vi "Test_Run All Tests.vi"(8 "error in":errorcluster, 9 "Modules":T7, 10 "Part Number 2":refnum<vi>, 11 "Test Selection":T8) -> (0 "error out":errorcluster)   [LabVIEW 2025]
uses:
  Controls/Test list.ctl
  Controls/tests tab control.ctl
  Controls/Graphs/XY Graph_Transparent.ctl
  Controls/Test Results/Test Pass Fail.ctl
  Controls/Test Results/Results Table.ctl
  Controls/Numeric Voltage.ctl
  Controls/Numeric Current.ctl
  SubVIs/Test_Calculate Wear-in.vi
  SubVIs/Test_Calculate Drop-out.vi
  SubVIs/Test_Calculate CRT.vi
  SubVIs/Test_Calculate Pull-in.vi
  SubVIs/Test_Calculate Hold-in.vi
  SubVIs/Test_Calculate ORT.vi
  Classes/Solenoid/Solenoid.lvclass
  Libraries/Power Supply/Power Supply.lvlib
  Libraries/USB IO/USB IO.lvlib
panel:
  out "Voltage Chart":dbl(graph)
  out "Current":T1 format="%5.3f A"
  out "Voltage":T2 format="%5.3f V"
  out "result 3":bool
  out "result 2":bool
  out "result":bool
  in  "Table Control":T3=[["Wear-in", "N/A", "N/A", "", "", "", "", ""], ["Drop-out", "N/A", "N/A", "", "", "", "", ""], ["Closing Response Time", "N/A", "N/A", "", "", "", "", ""], ["Pull-in", "N/A", "N/A", "", "", "", "", ""], ["Hold-in", "N/A", "N/A", "", "", "", "", ""], ["Opening Response Time", "N/A", "N/A", "", "", "", "", ""]]
  out "Errors":errorcluster
  in  "Tab Control":T4=enum."Wear-in"
  out "Power Supply Output":bool
  out "Cycles":dbl format="%3.0f of"
  out "Total Cycles":dbl format="%3.0f"
  out "Unit On?":bool
  in  "Abort":bool
  out "Drop-out Voltage":T2 format="%5.3f V"
  out "Drop-out Current":T1 format="%5.3f A"
  out "CRT Graph":T5
  out "Closing Response Time":dbl format="%5.3f ms"
  out "Pass? 2":T6 caption="Test Result"
  out "Pull-in Voltage":T2 format="%5.3f V"
  out "Pull-in Current":T1 format="%5.3f A"
  in  "Abort 2":bool
  out "XY Graph":T5
  out "Pass?":T6 caption="Test Result"
  out "Opening Response Time":dbl format="%5.3f ms"
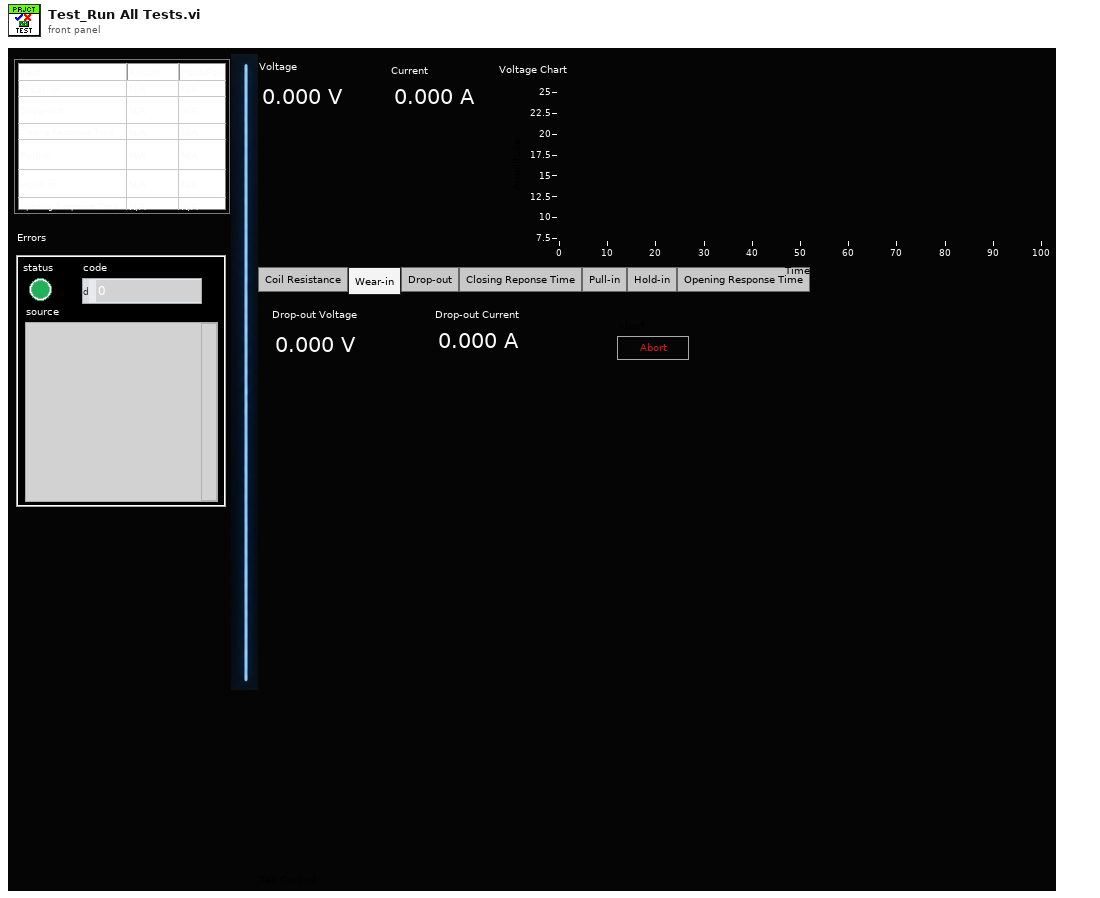
[diagram p1: front panel]
types:
  T1 = typedef "Numeric Current.ctl" = dbl
  T2 = typedef "Numeric Voltage.ctl" = dbl
  T3 = typedef "Results Table.ctl" = string[][]
  T4 = typedef "tests tab control.ctl" = enum32{"Coil Resistance", "Wear-in", "Drop-out", "Closing Reponse Time", "Pull-in", "Hold-in", "Opening Response Time"}
  T5 = typedef "XY Graph_Transparent.ctl" = cluster{dbl[], dbl[]}[]
  T6 = typedef "Test Pass Fail.ctl" = bool
  T7 = cluster{"Module IDs":i32[], "Module Names":string[]}
  T8 = typedef "Test list.ctl" = cluster{"Coil Resistance":bool, "Wear-in":bool, "Drop-out":bool, "Closing Response Time":bool, "Pull-in":bool, "Hold-in":bool, "Opening Response Time":bool}
  T9 = cluster{"V":dbl, "I":dbl, "Cycles":dbl, "On_Time_ms":dbl, "Off_Time_ms":dbl}
  T10 = cluster{"V":dbl, "I":dbl, "V_reduced":dbl, "V_perturb":dbl, "Plunger_Threshold":dbl, "Plunger_Threshold 2":dbl}
  T11 = cluster{"V":dbl, "I":dbl, "V_increased":dbl, "V_perturb":dbl, "Plunger_Threshold":dbl, "V_MAX":dbl}
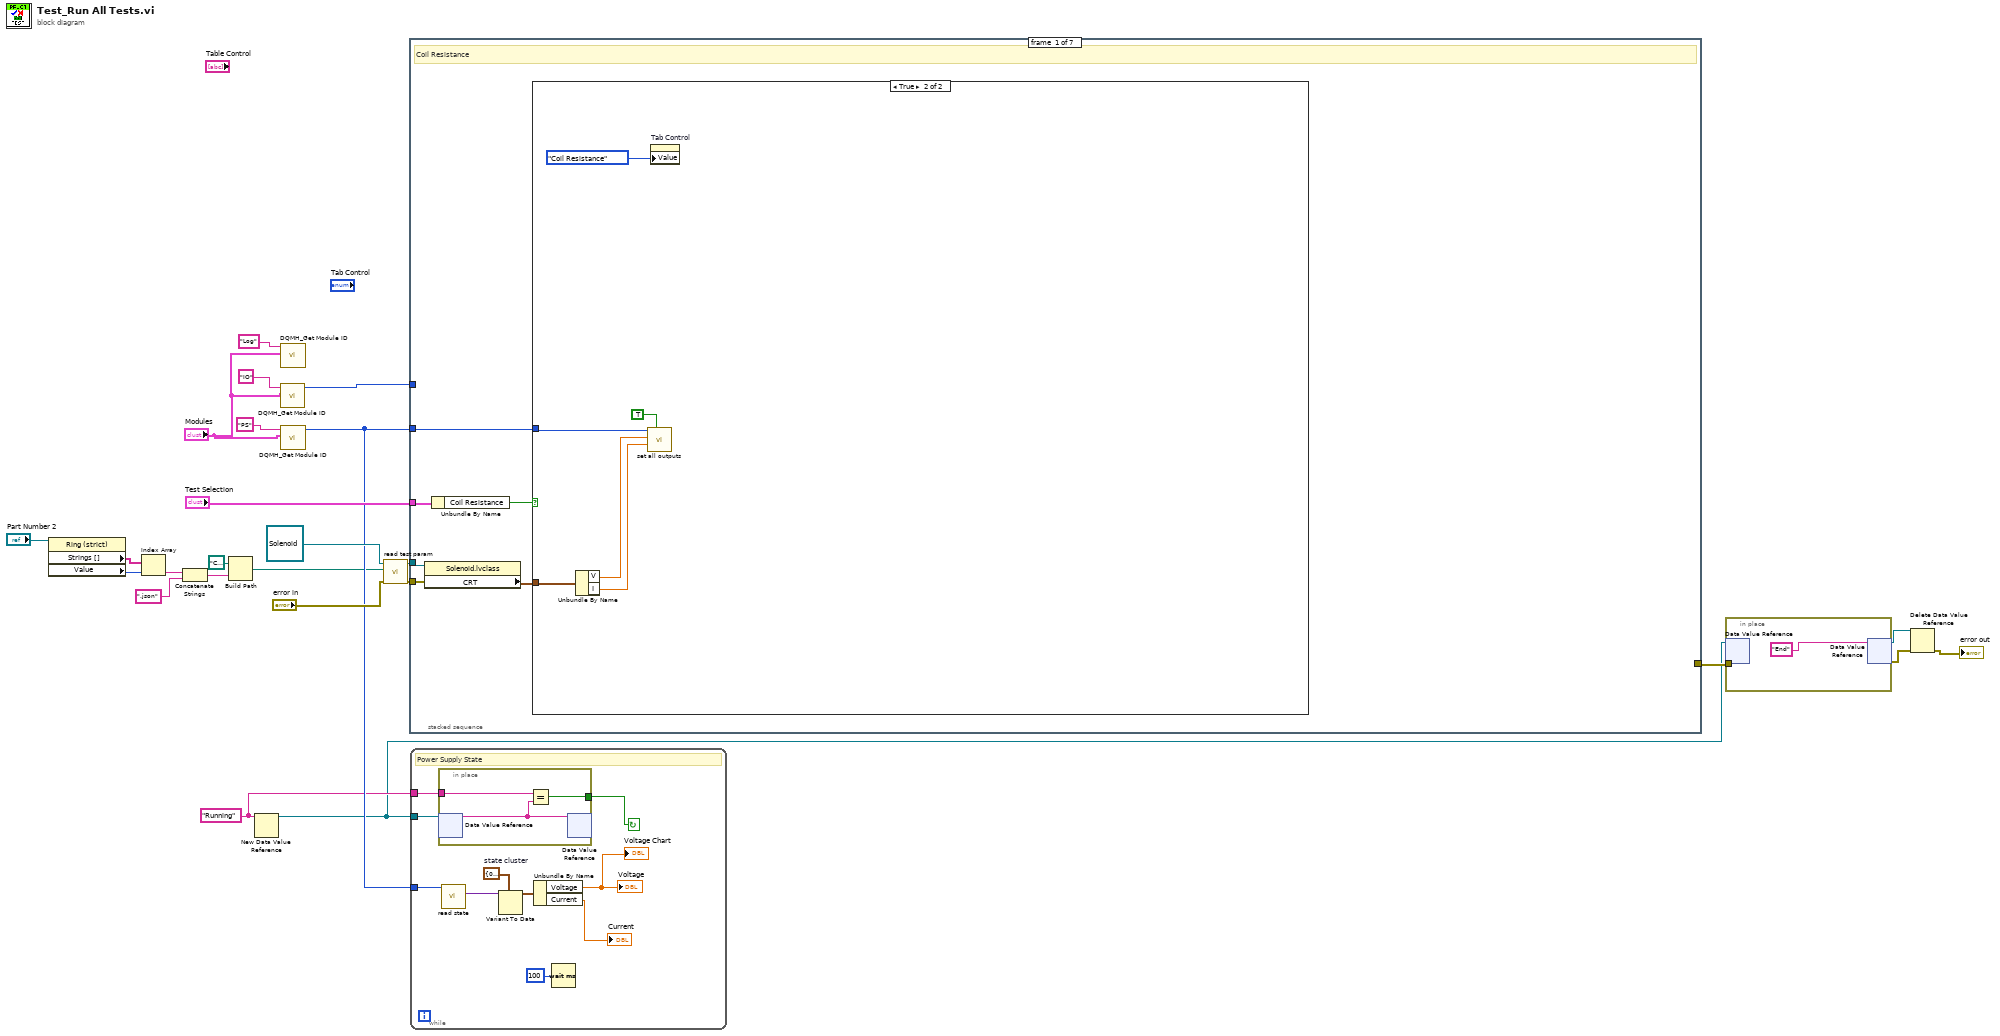
[diagram p0: block diagram]
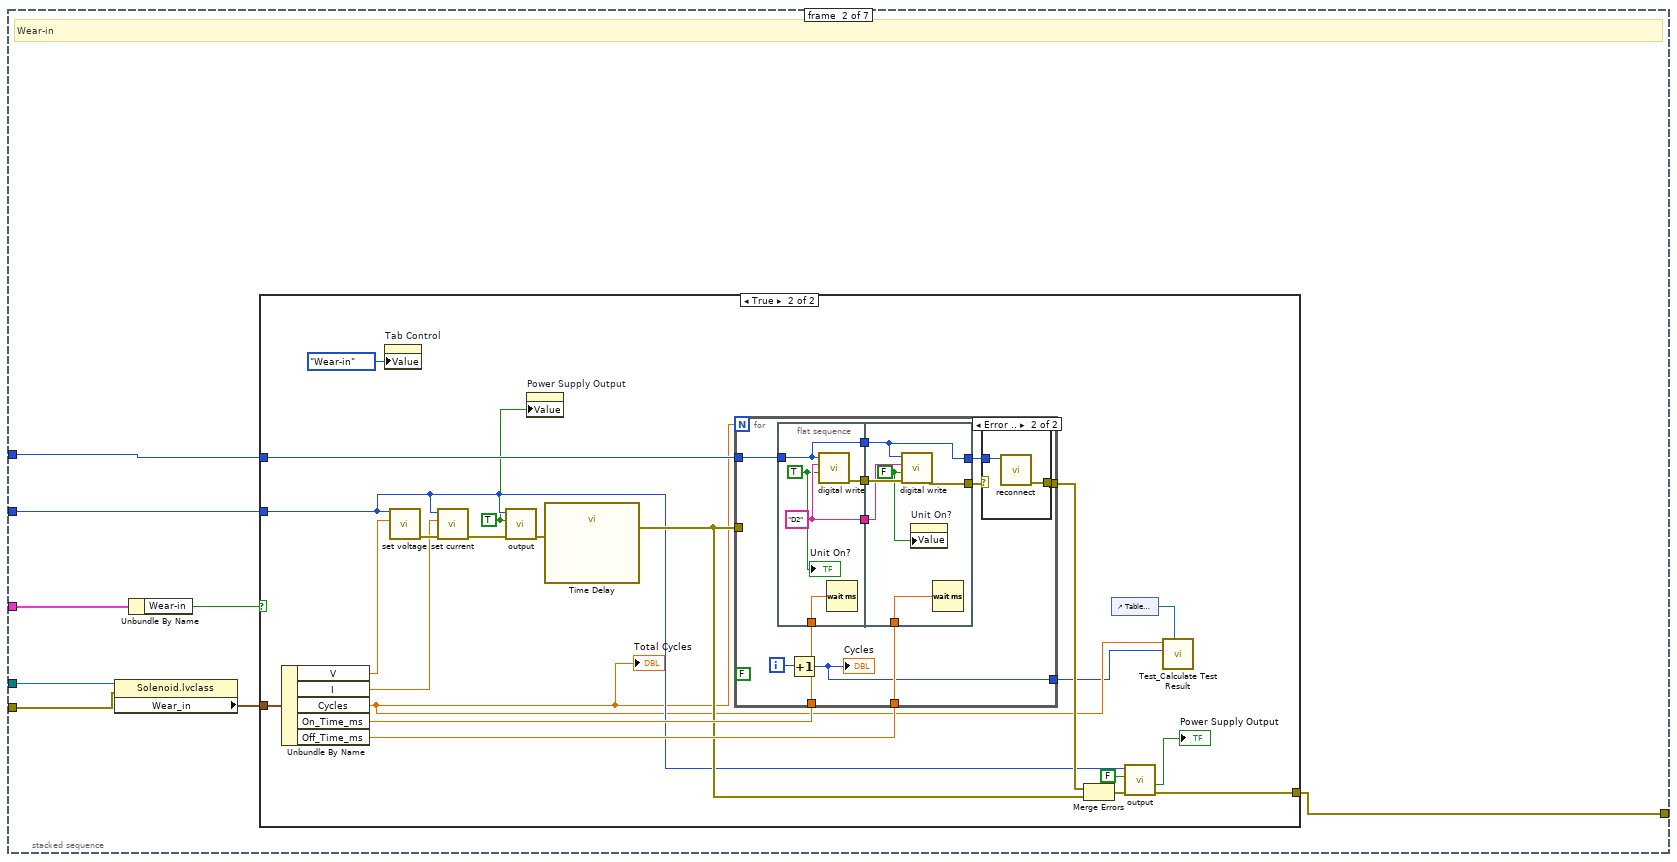
[diagram p3: hidden frame]
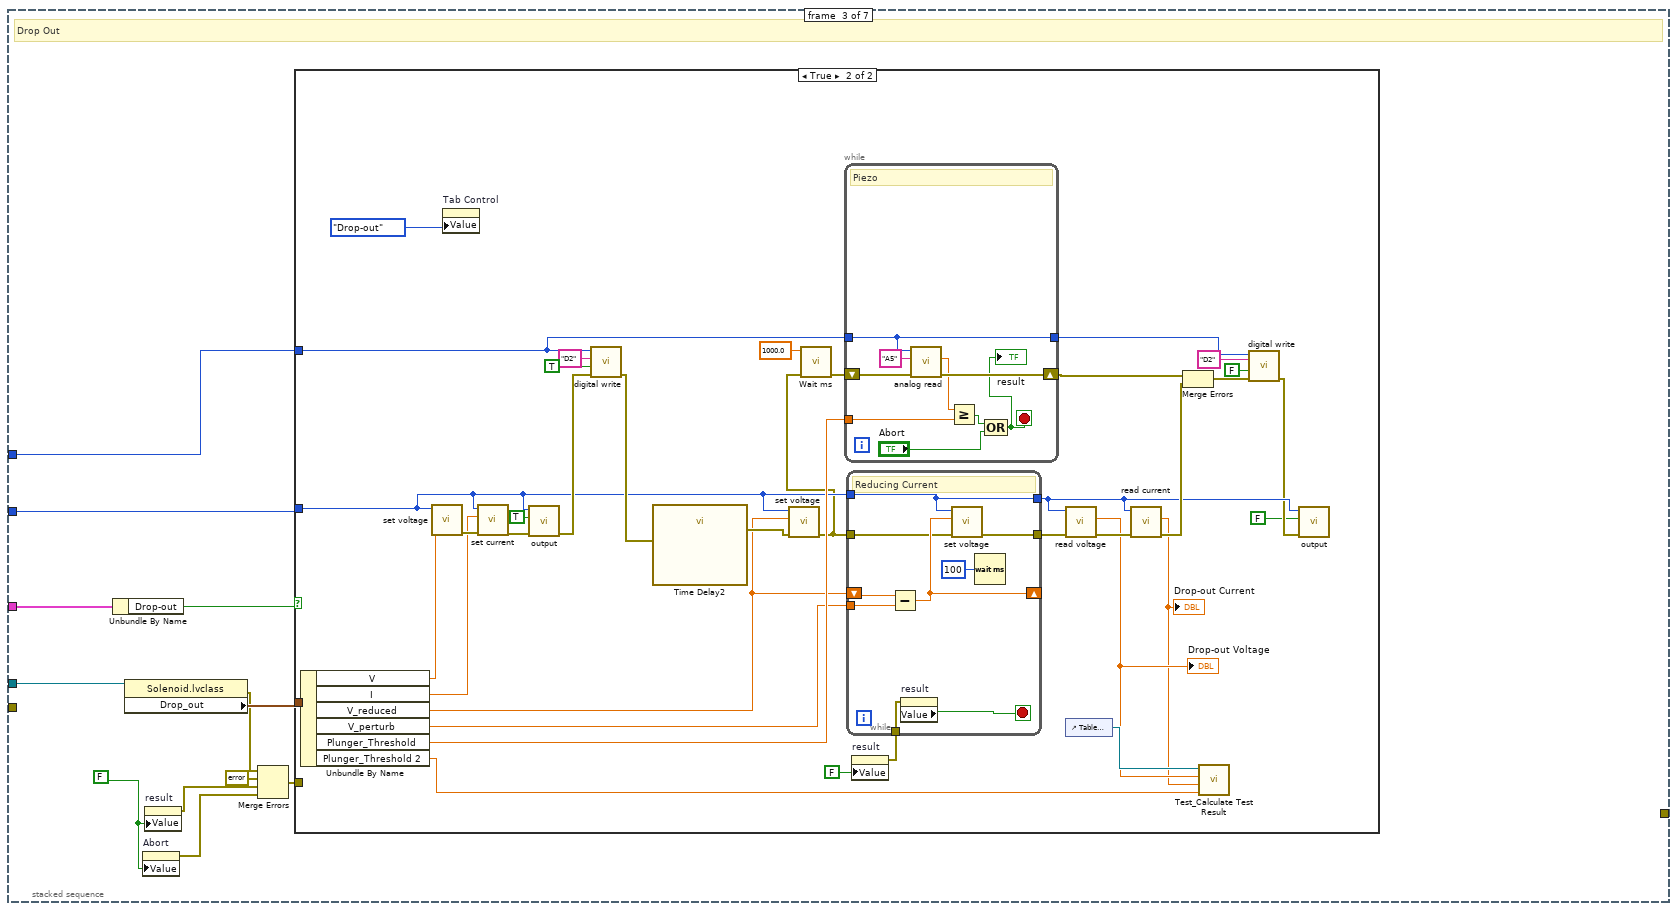
[diagram p6: hidden frame]
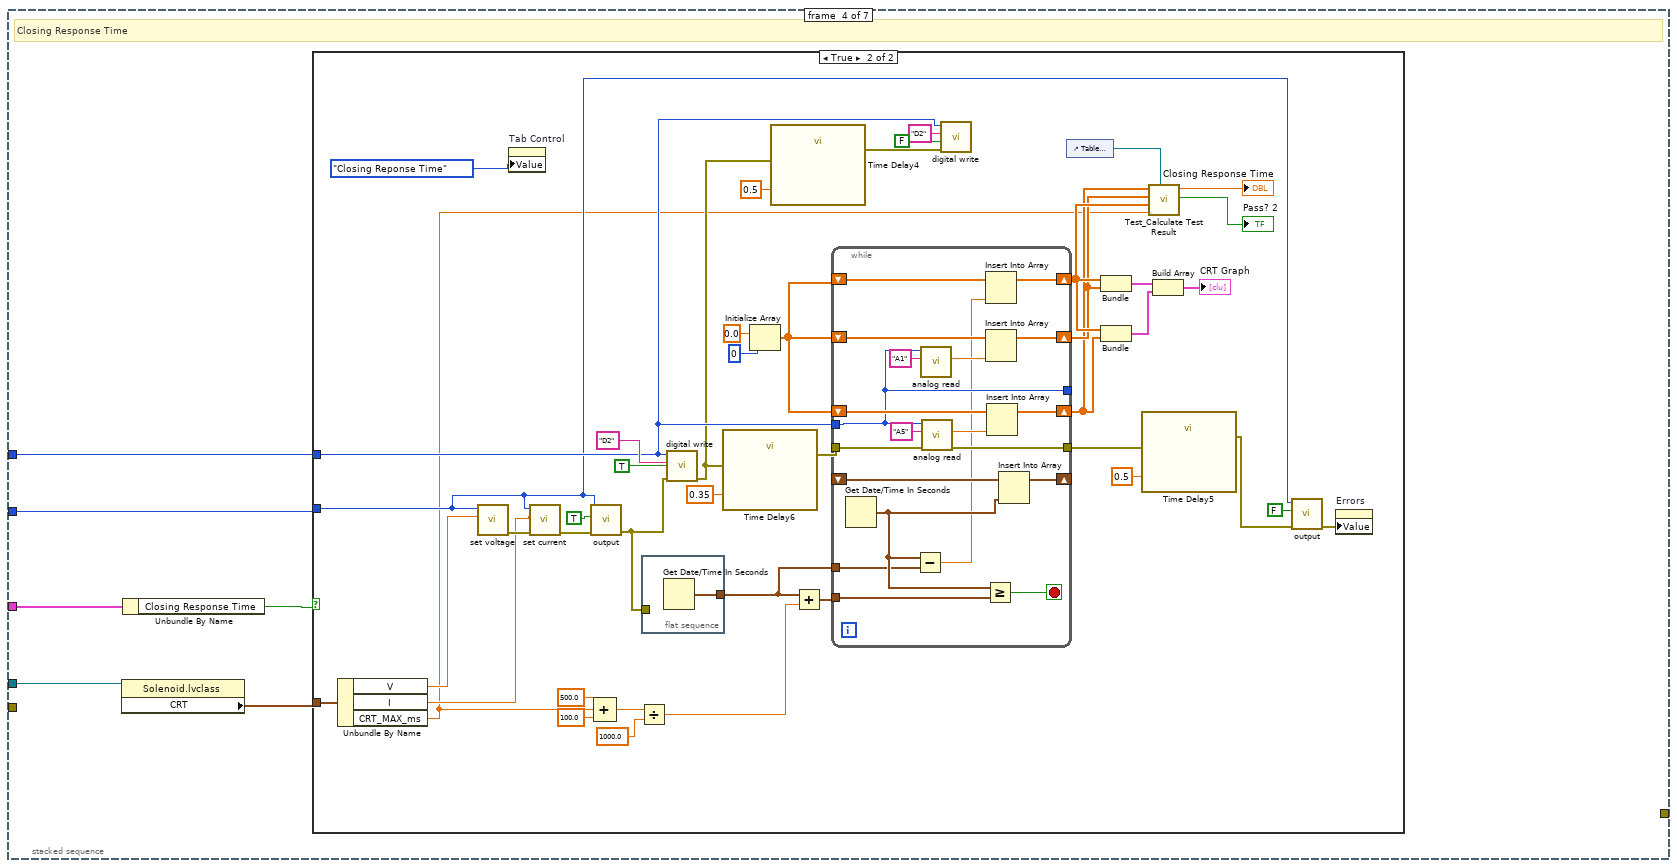
[diagram p8: hidden frame]
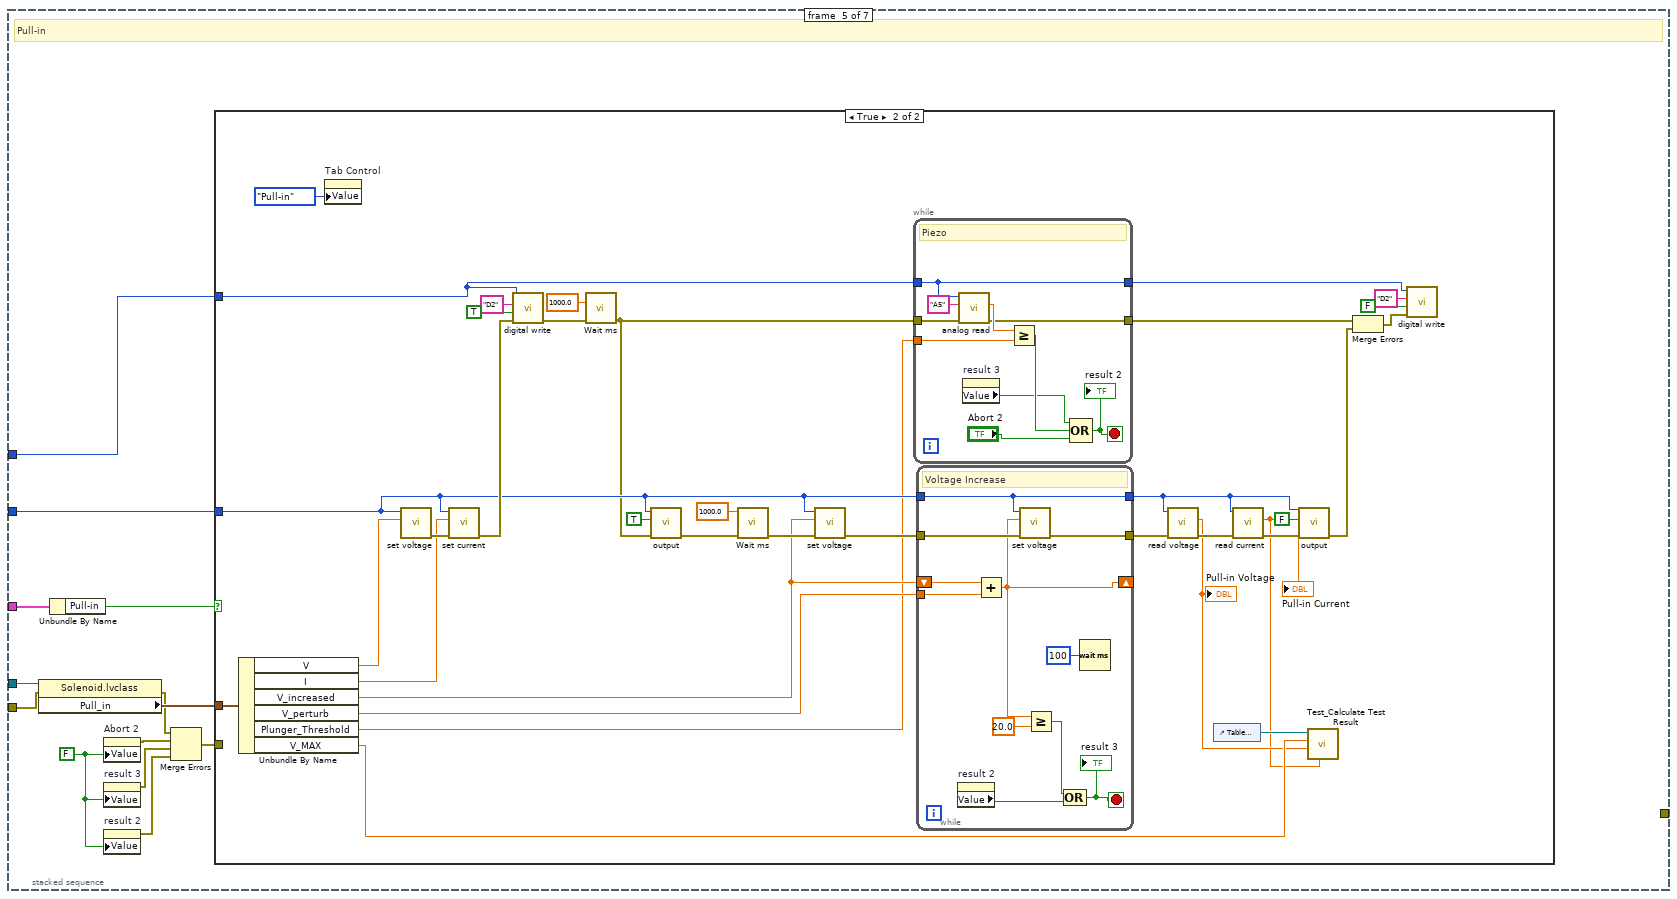
[diagram p10: hidden frame]
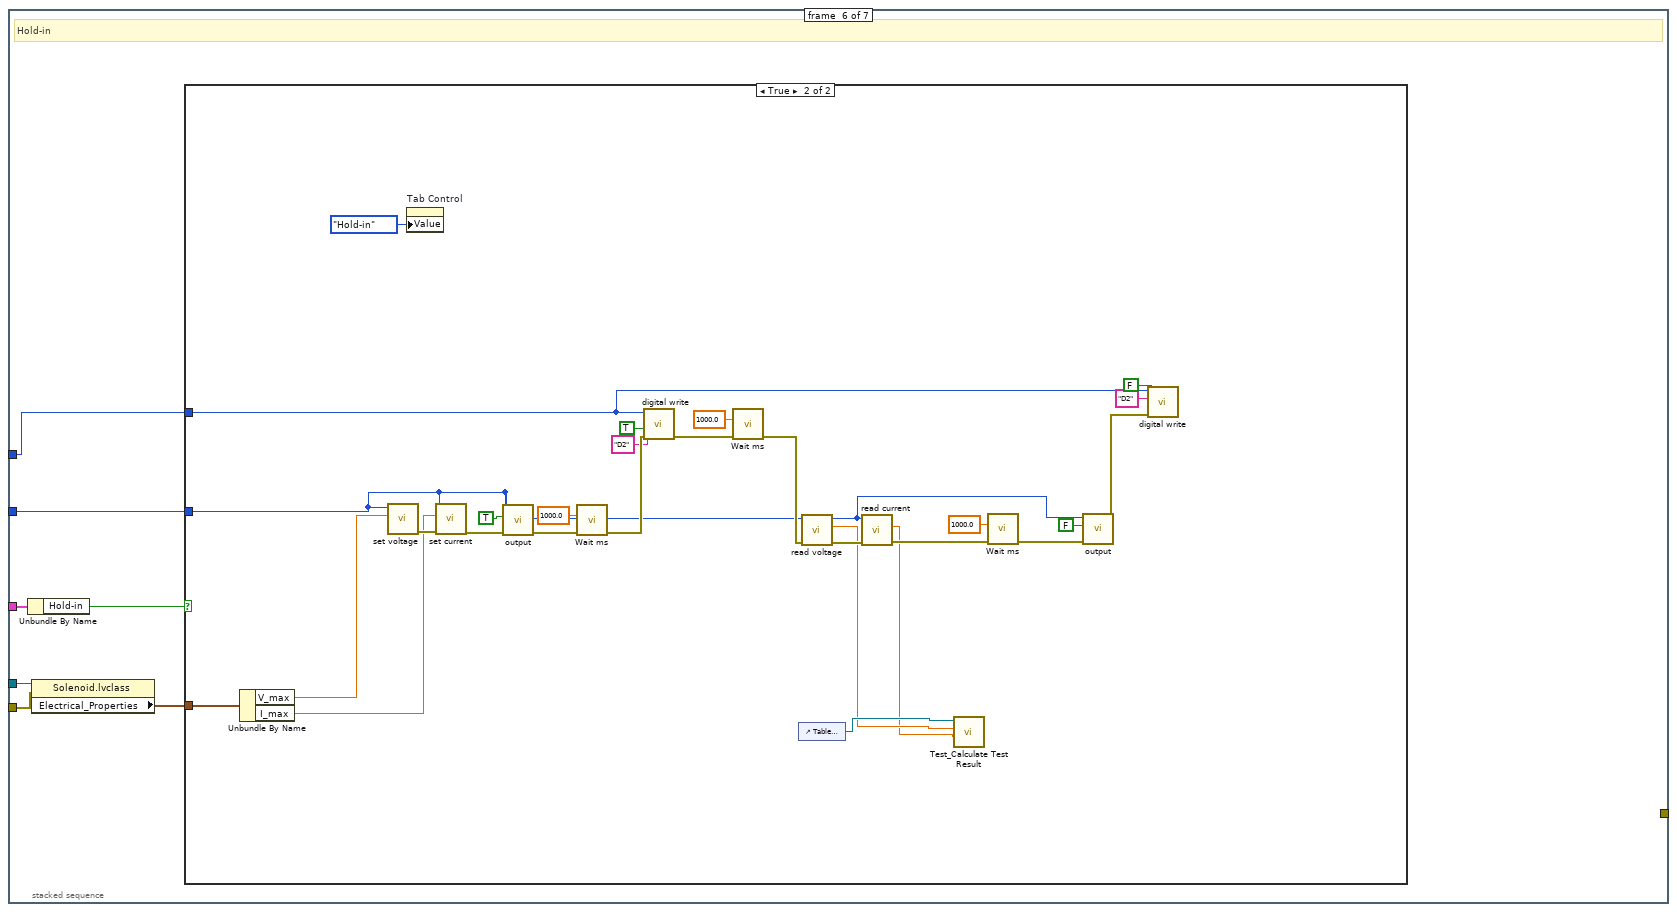
[diagram p12: hidden frame]
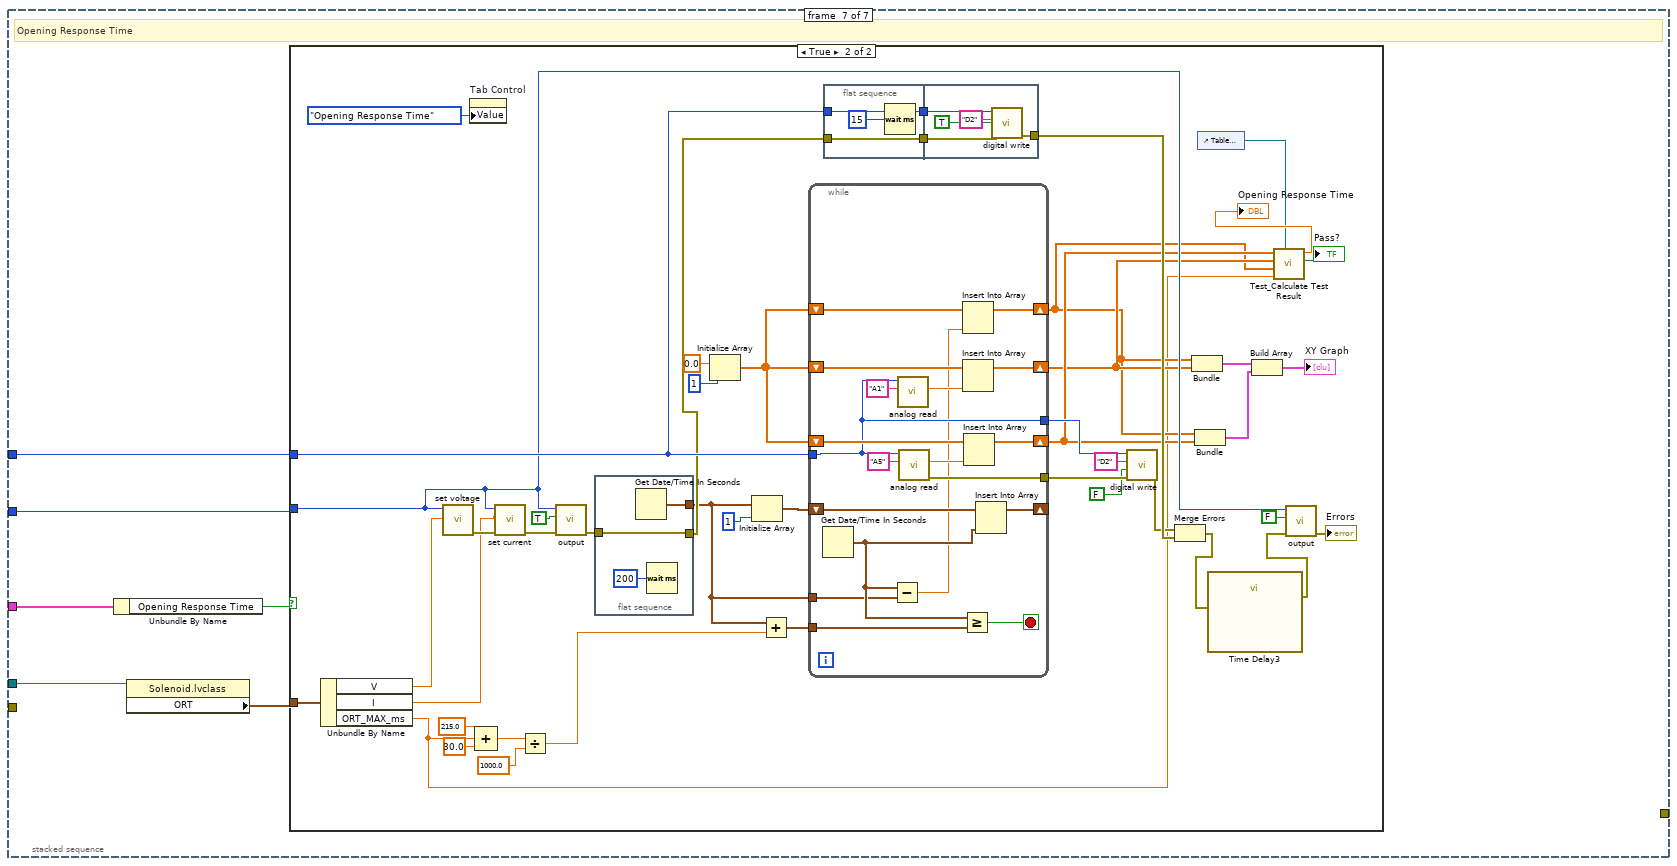
[diagram p14: hidden frame]
diagram:
  w14 = "Running"
  n1 = property class="Ring (strict)"(reference="Part Number 2") -> ("Strings []"=w7:string[], "Value"=w6:u16)  [unwired: 1 in, 2 out]
  n2 = Index Array(array=w7, index=w6) -> (element=w5:string)
  n3 = Concatenate Strings(w5, ".json" ("string")) -> (w3:string)
  n4 = Build Path(base path=path "C:/Users/Public/Documents/atp-station/programs", name or relative path=w3) -> (appended path=w1:path)
  n5 = New Data Value Reference(data value=w14) -> (data value reference=w12:refnum<data-value>)  [unwired: 1 in, 1 out]
  n6 = call "DQMH_Get Module ID.vi"("Modules"="Modules", "Module Name"="IO") -> ("Module ID out"=w16:i32)  [unwired: 9 in]
  n7 = call "DQMH_Get Module ID.vi"("Modules"="Modules", "Module Name"="Log") -> ()  [unwired: 9 in, 1 out]
  n8 = call "DQMH_Get Module ID.vi"("Modules"="Modules", "Module Name"="PS") -> ("Module ID out"=w15:i32)  [unwired: 9 in]
  n9 = call-dynamic "read test param.vi"("error in (no error)"="error in", "File Path"=w1, "Solenoid in"=refnum<class "Solenoid.lvclass"> refnum ("Solenoid.lvclass")) -> ("error out"=w21:errorcluster, "Solenoid out"=w23:refnum<class "Solenoid.lvclass">)  [unwired: 7 in]
  n10 = stacked-sequence {
    tunnel: w23 -> [w27 w43 w101 w162 w240 w304 w340]
    tunnel: "Test Selection" -> [w31 w45 w103 w164 w242 w306 w339]
    tunnel: w21 -> [w28 w42 _ _ w239 w303 _]
    tunnel: w15 -> [w29 w40 w99 w160 w237 w301 w336]
    tunnel: w16 -> [_ w39 w98 w159 w236 w300 w335]
    tunnel: [_ w38 _ _ _ _ _] -> w13
    frame #0 {
      # "Coil Resistance"
      n11 = property class="Solenoid.lvclass"(reference=w27, error in=w28) -> ("CRT"=w26:cluster{"V":dbl, "I":dbl, "CRT_MAX_ms":dbl})  [unwired: 2 out]
      n12 = Unbundle By Name(w31) -> ("Coil Resistance"=w30:bool)
      n13 = case shown="True" w30 {
        tunnel: w29 -> [_ w36]
        tunnel: w26 -> [_ w35]
        frame False {
        }
        frame True {
          n14 = Unbundle By Name(w35) -> ("V"=w33:dbl, "I"=w32:dbl)
          n15 = call "set all outputs.vi"("Output On/Off"=TRUE, "Current"=w32, "Voltage"=w33, "Module ID"=w36) -> ()  [unwired: 6 in, 2 out]
          n16 = property on="Tab Control" class="TabCtl (strict)"("Value"=tests_tab_control."Coil Resistance" ("Tab Control")) -> ()  [unwired: 2 in, 2 out]
        }
      }
    }
    frame #1 {
      # "Wear-in"
      n17 = property class="Solenoid.lvclass"(reference=w43, error in=w42) -> ("Wear_in"=w41:T9)  [unwired: 2 out]
      n18 = Unbundle By Name(w45) -> ("Wear-in"=w44:bool)
      n19 = case shown="True" w44 {
        tunnel: w41 -> [_ w66]
        tunnel: w40 -> [_ w55]
        tunnel: w39 -> [_ w62]
        tunnel: [_ w56] -> w38
        frame False {
        }
        frame True {
          w53 = TRUE ("Output On/Off")
          n20 = Unbundle By Name(w66) -> ("V"=w48:dbl, "I"=w47:dbl, "Cycles"=w51:dbl, "On_Time_ms"=w64:dbl, "Off_Time_ms"=w63:dbl)
          "Total Cycles" <- w51
          n21 = property on="Tab Control" class="TabCtl (strict)"("Value"=tests_tab_control."Wear-in" ("Tab Control")) -> ()  [unwired: 2 in, 2 out]
          n22 = call "set voltage.vi"("Output Voltage"=w48, "Module ID"=w55) -> ("error out"=w65:errorcluster)  [unwired: 8 in, 1 out]
          n23 = call "set current.vi"("error in"=w65, "Output Current"=w47, "Module ID"=w55) -> ("error out"=w61:errorcluster)  [unwired: 7 in, 1 out]
          n24 = call "output.vi"("error in"=w61, "Output On/Off"=w53, "Module ID"=w55) -> ("error out"=w60:errorcluster)  [unwired: 7 in, 1 out]
          n25 = property on="Power Supply Output" class="Bool (strict)"("Value"=w53) -> ()  [unwired: 2 in, 2 out]
          n26 = call "Time Delay"("error in (no error)"=w60) -> ("error out"=w58:errorcluster)  [unwired: 10 in]
          n27 = for {
            N: w51 -> [_]
            tunnel: w64 -> [w77]
            tunnel: w63 -> [w76]
            tunnel: w62 -> [w75]
            tunnel: w58 -> [_]
            tunnel: [w69] -> w59
            tunnel: [w67] -> w50
            i -> [w71]
            (unwired) FALSE ("Power Supply Output")
            n28 = flat-sequence {
              tunnel: w77 -> [w85]
              tunnel: w75 -> [w83]
              tunnel: [w84] -> w74
              tunnel: [w83] -> w73
              tunnel: [w82] -> w72
              tunnel: w76 -> [w89]
              tunnel: w74 -> [w91]
              tunnel: w73 -> [w86]
              tunnel: w72 -> [w90]
              tunnel: [w88] -> w70
              tunnel: [w86] -> w68
              frame #0 {
                w81 = TRUE ("On/Off")
                w82 = "D2" ("Line")
                n29 = call "digital write.vi"("On/Off"=w81, "Line"=w82, "Module ID"=w83) -> ("error out"=w84:errorcluster)  [unwired: 7 in, 1 out]
                n30 = Wait (ms)(milliseconds to wait=w85) -> ()  [unwired: 1 out]
                "Unit On?" <- w81
              }
              frame #1 {
                w87 = FALSE ("On/Off")
                n31 = call "digital write.vi"("error in"=w91, "On/Off"=w87, "Line"=w90, "Module ID"=w86) -> ("error out"=w88:errorcluster)  [unwired: 6 in, 1 out]
                n32 = property on="Unit On?" class="Bool (strict)"("Value"=w87) -> ()  [unwired: 2 in, 2 out]
                n33 = Wait (ms)(milliseconds to wait=w89) -> ()  [unwired: 1 out]
              }
            }
            n34 = Increment(x=w71) -> (x+1=w67:i32)
            "Cycles" <- w67
            n35 = case shown="Error .." w70 {
              selector: w70 -> [w78 _]
              tunnel: [w78 w80] -> w69
              tunnel: w68 -> [_ w79]
              frame No Error {
              }
              frame Error {
                n36 = call "reconnect.vi"("Module ID"=w79) -> ("error out"=w80:errorcluster)  [unwired: 9 in, 1 out]
              }
            }
          }
          n37 = Merge Errors(w59, w58) -> (w57:errorcluster)
          n38 = control-ref of="Table Control"() -> (w49:refnum<vi>)
          n39 = call "output.vi"("error in"=w57, "Output On/Off"=FALSE, "Module ID"=w55) -> ("error out"=w56:errorcluster, "timed out?"=→"Power Supply Output":bool)  [unwired: 7 in]
          n40 = call-poly "Test_Calculate Test Result.vi"("Table Ref"=w49, "Cycles"=w50, "Total Cycles"=w51) -> ()  [unwired: 7 in, 2 out]
        }
      }
    }
    frame #2 {
      w97 = FALSE
      # "Drop Out"
      n41 = Unbundle By Name(w103) -> ("Drop-out"=w102:bool)
      n42 = property class="Solenoid.lvclass"(reference=w101) -> (error out=w96:errorcluster, "Drop_out"=w100:T10)  [unwired: 1 in, 1 out]
      n43 = property on="Abort" class="Bool (strict)"("Value"=w97) -> (error out=w94:errorcluster)  [unwired: 2 in, 1 out]
      n44 = property on="result" class="Bool (strict)"("Value"=w97) -> (error out=w95:errorcluster)  [unwired: 2 in, 1 out]
      n45 = Merge Errors(w96, errorcluster {"status"=FALSE, "code"=0, "source"=""} ("error in"), w95, w94) -> (w93:errorcluster)
      n46 = case shown="True" w102 {
        tunnel: w100 -> [_ w140]
        tunnel: w99 -> [_ w127]
        tunnel: w98 -> [_ w131]
        tunnel: w93 -> [_ _]
        frame False {
        }
        frame True {
          n47 = Unbundle By Name(w140) -> ("V"=w106:dbl, "I"=w105:dbl, "V_reduced"=w129:dbl, "V_perturb"=w128:dbl, "Plunger_Threshold"=w130:dbl, "Plunger_Threshold 2"=w112:dbl)
          n48 = call "set voltage.vi"("Output Voltage"=w106, "Module ID"=w127) -> ("error out"=w139:errorcluster)  [unwired: 8 in, 1 out]
          n49 = property on="Tab Control" class="TabCtl (strict)"("Value"=tests_tab_control."Drop-out" ("Tab Control")) -> ()  [unwired: 2 in, 2 out]
          n50 = call "set current.vi"("error in"=w139, "Output Current"=w105, "Module ID"=w127) -> ("error out"=w138:errorcluster)  [unwired: 7 in, 1 out]
          n51 = call "output.vi"("error in"=w138, "Output On/Off"=TRUE, "Module ID"=w127) -> ("error out"=w136:errorcluster)  [unwired: 7 in, 1 out]
          n52 = call "digital write.vi"("error in"=w136, "On/Off"=TRUE, "Line"="D2", "Module ID"=w131) -> ("error out"=w132:errorcluster)  [unwired: 6 in, 1 out]
          n53 = call "Time Delay2"("error in (no error)"=w132) -> ("error out"=w133:errorcluster)  [unwired: 10 in]
          n54 = call "set voltage.vi"("error in"=w133, "Output Voltage"=w129, "Module ID"=w127) -> ("error out"=w110:errorcluster)  [unwired: 7 in, 1 out]
          n55 = call "Wait ms.vi"("error in (no error)"=w110, "Delay Time (ms)"=1000.0) -> ("error out"=w111:errorcluster)  [unwired: 9 in]
          n56 = while {
            tunnel: w131 -> [w154]
            shift-right: [w157] -> w124
            shift-left: w111 -> [w151]
            tunnel: w130 -> [w155]
            tunnel: [w154] -> w122
            stop <- w152 stop-if-true
            # "Piezo"
            n57 = call "analog read.vi"("error in"=w151, "Line"="A5", "Module ID"=w154) -> ("error out"=w157:errorcluster, "Voltage"=w156:T2)  [unwired: 6 in, 1 out]
            n58 = Greater Or Equal?(x=w156, y=w155) -> (x >= y?=w150:bool)
            n59 = Compound Arithmetic op=OR(w150, "Abort") -> (w152:bool)
            "result" <- w152
          }
          n60 = property on="result" class="Bool (strict)"("Value"=FALSE) -> (error out=w108:errorcluster)  [unwired: 2 in, 1 out]
          n61 = while {
            shift-right: [w144] -> _
            shift-left: w129 -> [w149]
            tunnel: w128 -> [w148]
            tunnel: w110 -> [w143]
            tunnel: w127 -> [w145]
            tunnel: [w147] -> w126
            tunnel: [w145] -> w119
            tunnel: w108 -> [w142]
            stop <- w141 stop-if-true
            # "Reducing Current"
            n62 = Subtract(x=w149, y=w148) -> (x-y=w144:dbl)
            n63 = property on="result" class="Bool (strict)"(error in=w142) -> ("Value"=w141:bool)  [unwired: 1 in, 2 out]
            n64 = call "set voltage.vi"("error in"=w143, "Output Voltage"=w144, "Module ID"=w145) -> ("error out"=w147:errorcluster)  [unwired: 7 in, 1 out]
            n65 = Wait (ms)(milliseconds to wait=u32 100) -> ()  [unwired: 1 out]
          }
          n66 = call "read voltage.vi"("error in"=w126, "Module ID"=w119) -> ("error out"=w125:errorcluster, "Volts"=w114:T2)  [unwired: 7 in, 1 out]
          "Drop-out Voltage" <- w114
          n67 = control-ref of="Table Control"() -> (w115:refnum<vi>)
          n68 = call "read current.vi"("error in"=w125, "Module ID"=w119) -> ("error out"=w123:errorcluster, "Amps"=w113:T1)  [unwired: 7 in, 1 out]
          "Drop-out Current" <- w113
          n69 = Merge Errors(w124, w123) -> (w118:errorcluster)
          n70 = call-poly "Test_Calculate Test Result.vi"("V_MIN"=w112, "Amps"=w113, "Volts"=w114, "Table in"=w115) -> ()  [unwired: 8 in]
          n71 = call "digital write.vi"("error in"=w118, "On/Off"=FALSE, "Line"="D2", "Module ID"=w122) -> ("error out"=w117:errorcluster)  [unwired: 6 in, 1 out]
          n72 = call "output.vi"("error in"=w117, "Output On/Off"=FALSE, "Module ID"=w119) -> ()  [unwired: 7 in, 2 out]
        }
      }
    }
    frame #3 {
      # "Closing Response Time"
      n73 = property class="Solenoid.lvclass"(reference=w162) -> ("CRT"=w161:cluster{"V":dbl, "I":dbl, "CRT_MAX_ms":dbl})  [unwired: 1 in, 2 out]
      n74 = Unbundle By Name(w164) -> ("Closing Response Time"=w163:bool)
      n75 = case shown="True" w163 {
        tunnel: w161 -> [_ w208]
        tunnel: w160 -> [_ w180]
        tunnel: w159 -> [_ w185]
        frame False {
        }
        frame True {
          n76 = Unbundle By Name(w208) -> ("V"=w203:dbl, "I"=w204:dbl, "CRT_MAX_ms"=w170:dbl)
          n77 = call "set voltage.vi"("Output Voltage"=w203, "Module ID"=w180) -> ("error out"=w207:errorcluster)  [unwired: 8 in, 1 out]
          n78 = property on="Tab Control" class="TabCtl (strict)"("Value"=tests_tab_control."Closing Reponse Time" ("Tab Control")) -> ()  [unwired: 2 in, 2 out]
          n79 = call "set current.vi"("error in"=w207, "Output Current"=w204, "Module ID"=w180) -> ("error out"=w205:errorcluster)  [unwired: 7 in, 1 out]
          n80 = call "output.vi"("error in"=w205, "Output On/Off"=TRUE, "Module ID"=w180) -> ("error out"=w200:errorcluster)  [unwired: 7 in, 1 out]
          n81 = Compound Arithmetic op=ADD(500.0 ("value"), w170, 100.0 ("value")) -> (w197:dbl)
          n82 = Divide(x=w197, y=1000.0) -> (x/y=w193:dbl)
          n83 = flat-sequence {
            tunnel: w200 -> [_]
            tunnel: [w209] -> w194
            frame #0 {
              n84 = Get Date/Time In Seconds() -> (seconds since 1Jan1904=w209:timestamp)
            }
          }
          n85 = call "digital write.vi"("error in"=w200, "On/Off"=TRUE, "Line"="D2", "Module ID"=w185) -> ("error out"=w175:errorcluster)  [unwired: 6 in, 1 out]
          n86 = call "Time Delay6"("error in (no error)"=w175, "Delay Time (s)"=0.35) -> ("error out"=w174:errorcluster)  [unwired: 9 in]
          n87 = Initialize Array(0.0 ("element"), 0 ("dimension size")) -> (w190:dbl[])
          n88 = call "Time Delay4"("error in (no error)"=w175, "Delay Time (s)"=0.5) -> ("error out"=w188:errorcluster)  [unwired: 9 in]
          n89 = Add(x=w194, y=w193) -> (x+y=w195:timestamp)
          n90 = while {
            shift-right: [w222] -> w172
            shift-left: w190 -> [w229]
            shift-right: [w227] -> w171
            shift-left: w190 -> [w226]
            tunnel: w185 -> [w220]
            tunnel: [w221] -> w184
            tunnel: [w220] -> _
            shift-right: [w218] -> _
            shift-left: _ -> [w219]
            tunnel: w195 -> [w215]
            shift-right: [w214] -> w173
            shift-left: w190 -> [w213]
            tunnel: w194 -> [w211]
            tunnel: w174 -> [w210]
            stop <- w217 stop-if-true
            n91 = Get Date/Time In Seconds() -> (seconds since 1Jan1904=w216:timestamp)
            n92 = Subtract(x=w216, y=w211) -> (x-y=w212:dbl)
            n93 = call "analog read.vi"("Line"="A1", "Module ID"=w220) -> ("Voltage"=w228:T2)  [unwired: 7 in, 2 out]
            n94 = call "analog read.vi"("error in"=w210, "Line"="A5", "Module ID"=w220) -> ("error out"=w221:errorcluster, "Voltage"=w225:T2)  [unwired: 6 in, 1 out]
            n95 = Greater Or Equal?(x=w216, y=w215) -> (x >= y?=w217:bool)
            n96 = Insert Into Array(array=w213, new element=w212) -> (w214:dbl[])  [unwired: 1 in]
            n97 = Insert Into Array(array=w229, new element=w228) -> (w222:dbl[])  [unwired: 1 in]
            n98 = Insert Into Array(array=w226, new element=w225) -> (w227:dbl[])  [unwired: 1 in]
            n99 = Insert Into Array(array=w219, new element=w216) -> (w218:timestamp[])  [unwired: 1 in]
          }
          n100 = call "digital write.vi"("error in"=w188, "On/Off"=FALSE, "Line"="D2", "Module ID"=w185) -> ()  [unwired: 6 in, 2 out]
          n101 = control-ref of="Table Control"() -> (w166:refnum<vi>)
          n102 = Bundle(w173, w172) -> (w178:cluster{dbl[], dbl[]})  [unwired: 1 in]
          n103 = Bundle(w173, w171) -> (w177:cluster{dbl[], dbl[]})  [unwired: 1 in]
          n104 = call "Time Delay5"("error in (no error)"=w184, "Delay Time (s)"=0.5) -> ("error out"=w182:errorcluster)  [unwired: 9 in]
          n105 = call-poly "Test_Calculate Test Result.vi"("Table Ref"=w166, "CRT_MAX"=w170, "Time Data"=w173, "Current Data"=w172, "Piezo Data"=w171) -> ("Pass?"=→"Pass? 2":bool, "CRT [ms]"=→"Closing Response Time":dbl)  [unwired: 5 in]
          n106 = Build Array(w178, w177) -> (→"CRT Graph":cluster{dbl[], dbl[]}[])
          n107 = call "output.vi"("error in"=w182, "Output On/Off"=FALSE, "Module ID"=w180) -> ("error out"=w179:errorcluster)  [unwired: 7 in, 1 out]
          n108 = property on="Errors" class="Clust (strict)"("Value"=w179) -> ()  [unwired: 2 in, 2 out]
        }
      }
    }
    frame #4 {
      w231 = FALSE
      # "Pull-in"
      n109 = property class="Solenoid.lvclass"(reference=w240, error in=w239) -> (error out=w235:errorcluster, "Pull_in"=w238:T11)  [unwired: 1 out]
      n110 = Unbundle By Name(w242) -> ("Pull-in"=w241:bool)
      n111 = property on="Abort 2" class="Bool (strict)"("Value"=w231) -> (error out=w234:errorcluster)  [unwired: 2 in, 1 out]
      n112 = property on="result 3" class="Bool (strict)"("Value"=w231) -> (error out=w233:errorcluster)  [unwired: 2 in, 1 out]
      n113 = property on="result 2" class="Bool (strict)"("Value"=w231) -> (error out=w232:errorcluster)  [unwired: 2 in, 1 out]
      n114 = Merge Errors(w235, w234, w233, w232) -> (w230:errorcluster)
      n115 = case shown="True" w241 {
        tunnel: w238 -> [_ w276]
        tunnel: w237 -> [_ w263]
        tunnel: w236 -> [_ w261]
        tunnel: w230 -> [_ _]
        frame False {
        }
        frame True {
          n116 = Unbundle By Name(w276) -> ("V"=w275:dbl, "I"=w244:dbl, "V_increased"=w266:dbl, "V_perturb"=w265:dbl, "Plunger_Threshold"=w260:dbl, "V_MAX"=w247:dbl)
          n117 = property on="Tab Control" class="TabCtl (strict)"("Value"=tests_tab_control."Pull-in" ("Tab Control")) -> ()  [unwired: 2 in, 2 out]
          n118 = call "set voltage.vi"("Output Voltage"=w275, "Module ID"=w263) -> ("error out"=w278:errorcluster)  [unwired: 8 in, 1 out]
          n119 = call "set current.vi"("error in"=w278, "Output Current"=w244, "Module ID"=w263) -> ("error out"=w272:errorcluster)  [unwired: 7 in, 1 out]
          n120 = call "digital write.vi"("error in"=w272, "On/Off"=TRUE, "Line"="D2", "Module ID"=w261) -> ("error out"=w271:errorcluster)  [unwired: 6 in, 1 out]
          n121 = call "Wait ms.vi"("error in (no error)"=w271, "Delay Time (ms)"=1000.0) -> ("error out"=w262:errorcluster)  [unwired: 9 in]
          n122 = call "output.vi"("error in"=w262, "Output On/Off"=TRUE, "Module ID"=w263) -> ("error out"=w269:errorcluster)  [unwired: 7 in, 1 out]
          n123 = call "Wait ms.vi"("error in (no error)"=w269, "Delay Time (ms)"=1000.0) -> ("error out"=w267:errorcluster)  [unwired: 9 in]
          n124 = call "set voltage.vi"("error in"=w267, "Output Voltage"=w266, "Module ID"=w263) -> ("error out"=w264:errorcluster)  [unwired: 7 in, 1 out]
          n125 = while {
            tunnel: w262 -> [w299]
            tunnel: w261 -> [w290]
            tunnel: w260 -> [w294]
            tunnel: [w291] -> w250
            tunnel: [w290] -> w249
            stop <- w297 stop-if-true
            # "Piezo"
            n126 = call "analog read.vi"("error in"=w299, "Line"="A5", "Module ID"=w290) -> ("error out"=w291:errorcluster, "Voltage"=w295:T2)  [unwired: 6 in, 1 out]
            n127 = property on="result 3" class="Bool (strict)"() -> ("Value"=w292:bool)  [unwired: 2 in, 2 out]
            n128 = Greater Or Equal?(x=w295, y=w294) -> (x >= y?=w293:bool)
            n129 = Compound Arithmetic op=OR(w292, w293, "Abort 2") -> (w297:bool)
            "result 2" <- w297
          }
          n130 = while {
            shift-right: [w279] -> _
            shift-left: w266 -> [w289]
            tunnel: w265 -> [w288]
            tunnel: w264 -> [w286]
            tunnel: w263 -> [w280]
            tunnel: [w281] -> w258
            tunnel: [w280] -> w256
            stop <- w284 stop-if-true
            # "Voltage Increase"
            n131 = property on="result 2" class="Bool (strict)"() -> ("Value"=w285:bool)  [unwired: 2 in, 2 out]
            n132 = Add(x=w289, y=w288) -> (x+y=w279:dbl)
            n133 = call "set voltage.vi"("error in"=w286, "Output Voltage"=w279, "Module ID"=w280) -> ("error out"=w281:errorcluster)  [unwired: 7 in, 1 out]
            n134 = Greater Or Equal?(x=w279, y=20.0) -> (x >= y?=w282:bool)
            n135 = Compound Arithmetic op=OR(w282, w285) -> (w284:bool)
            "result 3" <- w284
            n136 = Wait (ms)(milliseconds to wait=u32 100) -> ()  [unwired: 1 out]
          }
          n137 = call "read voltage.vi"("error in"=w258, "Module ID"=w256) -> ("error out"=w259:errorcluster, "Volts"=w246:T2)  [unwired: 7 in, 1 out]
          "Pull-in Voltage" <- w246
          n138 = control-ref of="Table Control"() -> (w248:refnum<vi>)
          n139 = call "read current.vi"("error in"=w259, "Module ID"=w256) -> ("error out"=w257:errorcluster, "Amps"=w245:T1)  [unwired: 7 in, 1 out]
          "Pull-in Current" <- w245
          n140 = call "output.vi"("error in"=w257, "Output On/Off"=FALSE, "Module ID"=w256) -> ("error out"=w251:errorcluster)  [unwired: 7 in, 1 out]
          n141 = call-poly "Test_Calculate Test Result.vi"("Amps"=w245, "Volts"=w246, "V_MAX"=w247, "Table in"=w248) -> ()  [unwired: 8 in]
          n142 = Merge Errors(w250, w251) -> (w252:errorcluster)
          n143 = call "digital write.vi"("error in"=w252, "On/Off"=FALSE, "Line"="D2", "Module ID"=w249) -> ()  [unwired: 6 in, 2 out]
        }
      }
    }
    frame #5 {
      # "Hold-in"
      n144 = Unbundle By Name(w306) -> ("Hold-in"=w305:bool)
      n145 = property class="Solenoid.lvclass"(reference=w304, error in=w303) -> ("Electrical_Properties"=w302:cluster{"V_max":dbl, "I_max":dbl})  [unwired: 2 out]
      n146 = case shown="True" w305 {
        tunnel: w302 -> [_ w334]
        tunnel: w301 -> [_ w316]
        tunnel: w300 -> [_ w313]
        frame False {
        }
        frame True {
          n147 = Unbundle By Name(w334) -> ("V_max"=w332:dbl, "I_max"=w331:dbl)
          n148 = call "set voltage.vi"("Output Voltage"=w332, "Module ID"=w316) -> ("error out"=w333:errorcluster)  [unwired: 8 in, 1 out]
          n149 = property on="Tab Control" class="TabCtl (strict)"("Value"=tests_tab_control."Hold-in" ("Tab Control")) -> ()  [unwired: 2 in, 2 out]
          n150 = call "set current.vi"("error in"=w333, "Output Current"=w331, "Module ID"=w316) -> ("error out"=w329:errorcluster)  [unwired: 7 in, 1 out]
          n151 = call "output.vi"("error in"=w329, "Output On/Off"=TRUE, "Module ID"=w316) -> ("error out"=w327:errorcluster)  [unwired: 7 in, 1 out]
          n152 = call "Wait ms.vi"("error in (no error)"=w327, "Delay Time (ms)"=1000.0) -> ("error out"=w326:errorcluster)  [unwired: 9 in]
          n153 = call "digital write.vi"("error in"=w326, "On/Off"=TRUE, "Line"="D2", "Module ID"=w313) -> ("error out"=w323:errorcluster)  [unwired: 6 in, 1 out]
          n154 = call "Wait ms.vi"("error in (no error)"=w323, "Delay Time (ms)"=1000.0) -> ("error out"=w321:errorcluster)  [unwired: 9 in]
          n155 = control-ref of="Table Control"() -> (w310:refnum<vi>)
          n156 = call "read voltage.vi"("error in"=w321, "Module ID"=w316) -> ("error out"=w320:errorcluster, "Volts"=w309:T2)  [unwired: 7 in, 1 out]
          n157 = call "read current.vi"("error in"=w320, "Module ID"=w316) -> ("error out"=w319:errorcluster, "Amps"=w308:T1)  [unwired: 7 in, 1 out]
          n158 = call-poly "Test_Calculate Test Result.vi"("Amps"=w308, "Volts"=w309, "Table in"=w310) -> ()  [unwired: 9 in]
          n159 = call "Wait ms.vi"("error in (no error)"=w319, "Delay Time (ms)"=1000.0) -> ("error out"=w317:errorcluster)  [unwired: 9 in]
          n160 = call "output.vi"("error in"=w317, "Output On/Off"=FALSE, "Module ID"=w316) -> ("error out"=w314:errorcluster)  [unwired: 7 in, 1 out]
          n161 = call "digital write.vi"("error in"=w314, "On/Off"=FALSE, "Line"="D2", "Module ID"=w313) -> ()  [unwired: 6 in, 2 out]
        }
      }
    }
    frame #6 {
      # "Opening Response Time"
      n162 = Unbundle By Name(w339) -> ("Opening Response Time"=w338:bool)
      n163 = property class="Solenoid.lvclass"(reference=w340) -> ("ORT"=w337:cluster{"V":dbl, "I":dbl, "ORT_MAX_ms":dbl})  [unwired: 1 in, 2 out]
      n164 = case shown="True" w338 {
        tunnel: w337 -> [_ w385]
        tunnel: w336 -> [_ w362]
        tunnel: w335 -> [_ w366]
        frame False {
        }
        frame True {
          n165 = Unbundle By Name(w385) -> ("V"=w346:dbl, "I"=w345:dbl, "ORT_MAX_ms"=w347:dbl)
          n166 = call "set voltage.vi"("Output Voltage"=w346, "Module ID"=w362) -> ("error out"=w384:errorcluster)  [unwired: 8 in, 1 out]
          n167 = property on="Tab Control" class="TabCtl (strict)"("Value"=tests_tab_control."Opening Response Time" ("Tab Control")) -> ()  [unwired: 2 in, 2 out]
          n168 = Compound Arithmetic op=ADD(215.0 ("value"), w347, 30.0 ("value")) -> (w371:dbl)
          n169 = call "set current.vi"("error in"=w384, "Output Current"=w345, "Module ID"=w362) -> ("error out"=w382:errorcluster)  [unwired: 7 in, 1 out]
          n170 = Divide(x=w371, y=1000.0) -> (x/y=w368:dbl)
          n171 = call "output.vi"("error in"=w382, "Output On/Off"=TRUE, "Module ID"=w362) -> ("error out"=w369:errorcluster)  [unwired: 7 in, 1 out]
          n172 = flat-sequence {
            tunnel: [w396] -> w351
            tunnel: w369 -> [w395]
            tunnel: [w395] -> w364
            frame #0 {
              n173 = Get Date/Time In Seconds() -> (seconds since 1Jan1904=w396:timestamp)
              n174 = Wait (ms)(milliseconds to wait=u32 200) -> ()  [unwired: 1 out]
            }
          }
          n175 = Initialize Array(0.0 ("element"), 1 ("dimension size")) -> (w355:dbl[])
          n176 = Initialize Array(w351, 1 ("dimension size")) -> (w374:timestamp[])
          n177 = Add(x=w351, y=w368) -> (x+y=w367:timestamp)
          n178 = while {
            shift-right: [w408] -> w349
            shift-left: w355 -> [w415]
            shift-right: [w413] -> w350
            shift-left: w355 -> [w412]
            tunnel: w366 -> [w406]
            tunnel: [w407] -> w379
            tunnel: [w406] -> w378
            shift-right: [w404] -> _
            shift-left: w374 -> [w405]
            tunnel: w367 -> [w401]
            shift-right: [w400] -> w348
            shift-left: w355 -> [w399]
            tunnel: w351 -> [w397]
            stop <- w403 stop-if-true
            n179 = Get Date/Time In Seconds() -> (seconds since 1Jan1904=w402:timestamp)
            n180 = Subtract(x=w402, y=w397) -> (x-y=w398:dbl)
            n181 = call "analog read.vi"("Line"="A1", "Module ID"=w406) -> ("Voltage"=w414:T2)  [unwired: 7 in, 2 out]
            n182 = call "analog read.vi"("Line"="A5", "Module ID"=w406) -> ("error out"=w407:errorcluster, "Voltage"=w411:T2)  [unwired: 7 in, 1 out]
            n183 = Greater Or Equal?(x=w402, y=w401) -> (x >= y?=w403:bool)
            n184 = Insert Into Array(array=w399, new element=w398) -> (w400:dbl[])  [unwired: 1 in]
            n185 = Insert Into Array(array=w415, new element=w414) -> (w408:dbl[])  [unwired: 1 in]
            n186 = Insert Into Array(array=w412, new element=w411) -> (w413:dbl[])  [unwired: 1 in]
            n187 = Insert Into Array(array=w405, new element=w402) -> (w404:timestamp[])  [unwired: 1 in]
          }
          n188 = flat-sequence {
            tunnel: w366 -> [w388]
            tunnel: [w388] -> w365
            tunnel: w364 -> [w386]
            tunnel: [w386] -> w363
            tunnel: w365 -> [w391]
            tunnel: w363 -> [w390]
            tunnel: [w389] -> w361
            frame #0 {
              n189 = Wait (ms)(milliseconds to wait=u32 15) -> ()  [unwired: 1 out]
            }
            frame #1 {
              n190 = call "digital write.vi"("error in"=w390, "On/Off"=TRUE, "Line"="D2", "Module ID"=w391) -> ("error out"=w389:errorcluster)  [unwired: 6 in, 1 out]
            }
          }
          n191 = call "digital write.vi"("error in"=w379, "On/Off"=FALSE, "Line"="D2", "Module ID"=w378) -> ("error out"=w360:errorcluster)  [unwired: 6 in, 1 out]
          n192 = Merge Errors(w360, w361) -> (w357:errorcluster)
          n193 = Bundle(w348, w349) -> (w354:cluster{dbl[], dbl[]})  [unwired: 1 in]
          n194 = Bundle(w348, w350) -> (w353:cluster{dbl[], dbl[]})  [unwired: 1 in]
          n195 = control-ref of="Table Control"() -> (w342:refnum<vi>)
          n196 = call "Time Delay3"("error in (no error)"=w357) -> ("error out"=w356:errorcluster)  [unwired: 10 in]
          n197 = Build Array(w354, w353) -> (→"XY Graph":cluster{dbl[], dbl[]}[])
          n198 = call-poly "Test_Calculate Test Result.vi"("Table Ref"=w342, "ORT_MAX"=w347, "Time Data"=w348, "Current Data"=w349, "Piezo Data"=w350) -> ("Pass?"=→"Pass?":bool, "ORT [ms]"=→"Opening Response Time":dbl)  [unwired: 5 in]
          n199 = call "output.vi"("error in"=w356, "Output On/Off"=FALSE, "Module ID"=w362) -> ("error out"=→"Errors":errorcluster)  [unwired: 7 in, 1 out]
        }
      }
    }
  }
  n200 = while {
    tunnel: w15 -> [w425]
    tunnel: w12 -> [w419]
    tunnel: w14 -> [w418]
    stop <- w417 continue-if-true
    w423 = cluster{"Voltage":dbl, "Current":dbl} {"Voltage"=0.0, "Current"=0.0}  # state cluster
    # "Power Supply State"
    n201 = in-place {
      in-place-border: w418 -> [w427]
      in-place-border: [w426] -> w417
      n202 = in-place-dvr #1(w419) -> (w428:string)  [unwired: 1 out]
      n203 = Equal?(x=w427, y=w428) -> (x = y?=w426:bool)
      n204 = in-place-dvr #1(w428) -> ()  [unwired: 2 out]
    }
    n205 = call "read state.vi"("Module ID"=w425) -> ("Variant"=w424:variant)  [unwired: 8 in, 2 out]
    n206 = Variant To Data(type=w423, Variant=w424) -> (data=w422:cluster{"Voltage":dbl, "Current":dbl})  [unwired: 1 in, 1 out]
    n207 = Unbundle By Name(w422) -> ("Voltage"=→"Voltage" →"Voltage Chart":dbl, "Current"=→"Current":dbl)
    n208 = Wait (ms)(milliseconds to wait=u32 100) -> ()  [unwired: 1 out]
  }
  n209 = in-place {
    in-place-border: w13 -> [_]
    n210 = in-place-dvr #2(w12) -> ()  [unwired: 2 out]
    n211 = in-place-dvr #2("End") -> (w10:refnum<data-value>, w11:errorcluster)
  }
  n212 = Delete Data Value Reference(data value reference=w10, error in=w11) -> (error out=→"error out":errorcluster)  [unwired: 1 out]
